vi "Connection.vi"(8 "error in (no error)":errorcluster, 11 "TCPResource in":refnum<class "TCPResource.lvclass">) -> (0 "error out":errorcluster, 2 "Connection":refnum<class "Connection.lvclass">, 3 "TCPResource out":refnum<class "TCPResource.lvclass">)   [LabVIEW 2020, in "PicoG-Core.lvlib" / "TCPResource.lvclass"]
uses:
  TCPResource.lvclass
  <vilib>/IlluminatedG/lv-stream/Connection/Connection.lvclass
  TCPResource.lvclass/TCPResource.ctl
  <vilib>/IlluminatedG/lv-stream-tcp/TCP Client/TCP Client.lvclass
  C:/Program Files (x86)/National Instruments/LabVIEW 2020/vi.lib/IlluminatedG/lv-stream/Connection/Connection.lvclass
  C:/Program Files (x86)/National Instruments/LabVIEW 2020/vi.lib/IlluminatedG/lv-stream/Endpoint/Endpoint.lvclass
  C:/Program Files (x86)/National Instruments/LabVIEW 2020/vi.lib/IlluminatedG/lv-stream-tcp/TCP Client/TCP Client.lvclass
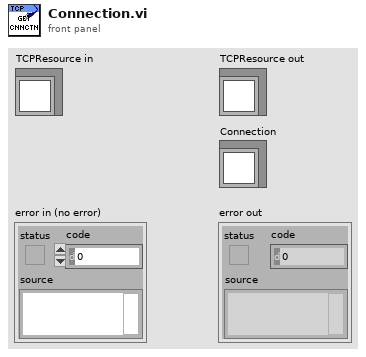
[diagram p1: front panel]
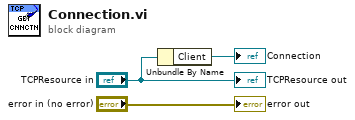
[diagram p0: block diagram]
diagram:
  n1 = Unbundle By Name("TCPResource in") -> ("Client"=→"Connection":refnum<class "TCP Client.lvclass">)
  "error out" <- "error in (no error)"
  "TCPResource out" <- "TCPResource in"
